vi "Image display-Set palette.vi"(8 "error in (no error)":errorcluster, 9 "Image Palette":refnum<vi>, 11 "Image Display":T1) -> (0 "error out":errorcluster, 3 "Image Display":T1)   [LabVIEW 2020]
uses:
  Typedefs/Image display ref.ctl
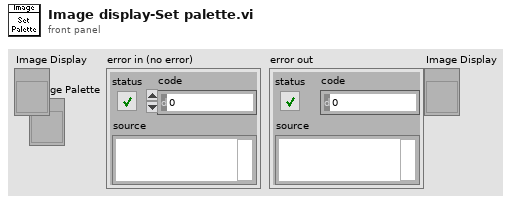
[diagram p1: front panel]
types:
  T1 = typedef "Image display ref.ctl" = refnum<vi>
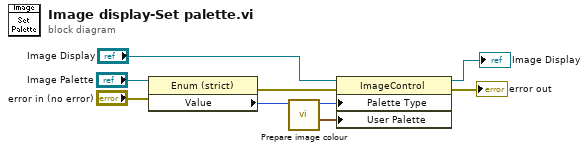
[diagram p0: block diagram]
diagram:
  n1 = property class="Enum (strict)"(reference="Image Palette", error in="error in (no error)") -> (error out=w5:errorcluster, "Value"=w9:enum16{"Gray", "Red", "Green"})  [unwired: 1 out]
  n2 = call "Prepare image colour.vi"("Left Image Palette"=w9) -> ("Color Palette"=w6:cluster{"Red":u8, "Green":u8, "Blue":u8}[], "Palette Type"=w7:u32)  [unwired: 8 in, 1 out]
  n3 = property on="Property Node" class="ImageControl"(reference="Image Display", error in=w5, "Palette Type"=w7, "User Palette"=w6) -> (reference out=→"Image Display":T1, error out=→"error out":errorcluster)
